vi "Config.vi"(7 "Open (T)":bool=TRUE, 8 "error in (no error)":errorcluster, 11 "COM PPORT":refnum<visa-resource-name>) -> (0 "error out":errorcluster, 3 "refnum out":refnum<visa-resource-name>)   [LabVIEW 2020, in "Korad KA3305P.lvlib"]
uses:
  Korad KA3305P.lvlib
  <vilib>/Instr/_visa.llb/VISA Configure Serial Port (Instr).vi
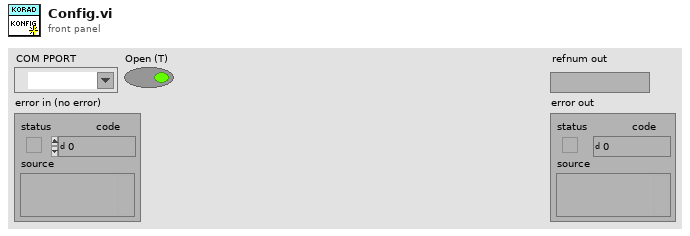
[diagram p1: front panel]
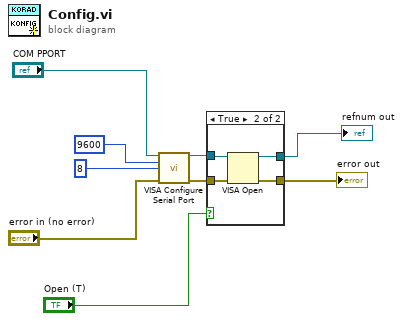
[diagram p0: block diagram]
diagram:
  n1 = call-poly "VISA Configure Serial Port"("VISA resource name"="COM PPORT", "baud rate (9600)"=u32 9600, "data bits (8)"=u16 8, "error in (no error)"="error in (no error)") -> ("VISA resource name out"=w5:refnum<visa-resource-name>, "error out"=w4:errorcluster)  [unwired: 10 in]
  n2 = case shown="True" "Open (T)" {
    tunnel: w5 -> [w11 w15]
    tunnel: w4 -> [w10 w14]
    tunnel: [w10 w13] -> w3
    tunnel: [w11 w12] -> w2
    frame False {
    }
    frame True {
      n3 = VISA Open(error in (no error)=w14, VISA resource name=w15) -> (VISA resource name=w12:refnum<visa-resource-name>, error out=w13:errorcluster)  [unwired: 3 in]
    }
  }
  "refnum out" <- w2
  "error out" <- w3
